vi "main.vi"() -> ()   [LabVIEW 2019]
uses:
  Program Files (x86)/SimpleLibrary/SimpleLib.dll
panel:
  in  "Exit":bool
  in  "OK":bool
  in  "Message to display":string
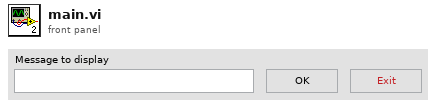
[diagram p1: front panel]
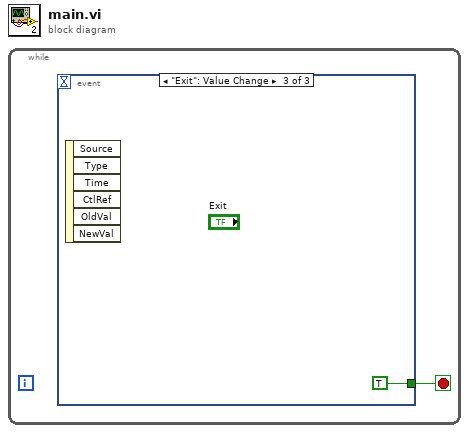
[diagram p0: block diagram]
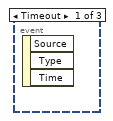
[diagram p2: hidden frame]
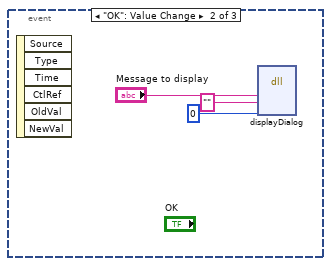
[diagram p3: hidden frame]
diagram:
  n1 = while {
    stop <- w1 stop-if-true
    n2 = event shown="[2] \"Exit\": Value Change" {
      selector: _ -> [_ _ _]
      dyn-events: _ -> [_ _ _]
      timeout: _ -> [_ _ _]
      tunnel: [_ _ TRUE] -> w1
      event Timeout {
        n3 = event-data() -> ()  [unwired: 1 in, 3 out]
      }
      event "OK": Value Change {
        n4 = event-data() -> ()  [unwired: 1 in, 6 out]
        n5 = dll-call lib="C:/Program Files (x86)/SimpleLibrary/SimpleLib.dll" fn="displayDialog"("StringIn"="Message to display", "StringOut"="", "len"=0) -> ()  [unwired: 7 in, 2 out]
      }
      event "Exit": Value Change {
        n6 = event-data() -> ()  [unwired: 1 in, 6 out]
      }
    }
  }
